vi "Test Component A Does Something.vi"(11 "Test Case In":refnum<class "Some Component A Test.lvclass">) -> (0 "error out":errorcluster, 3 "Test Case Out":refnum<class "Some Component A Test.lvclass">)   [LabVIEW 2020, in "Component A Test Suite.lvlib" / "Some Component A Test.lvclass"]
uses:
  Some Component A Test.lvclass
  Some Component A Test.lvclass/Some Component A Test.ctl
  b08caf3d-bad9-44fb-9ac4-9cc6f929a6d7.vi
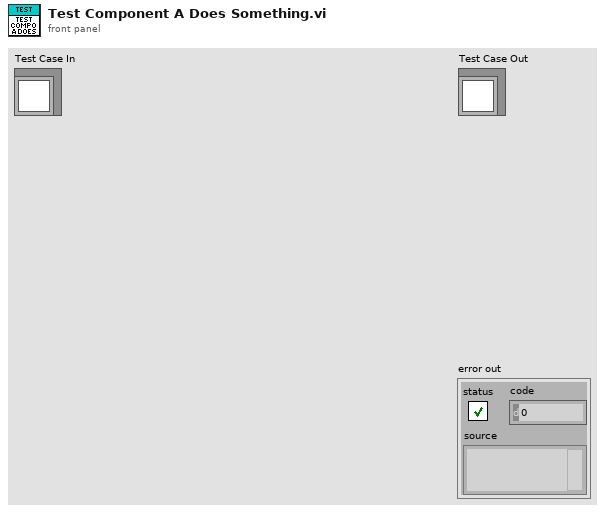
[diagram p1: front panel]
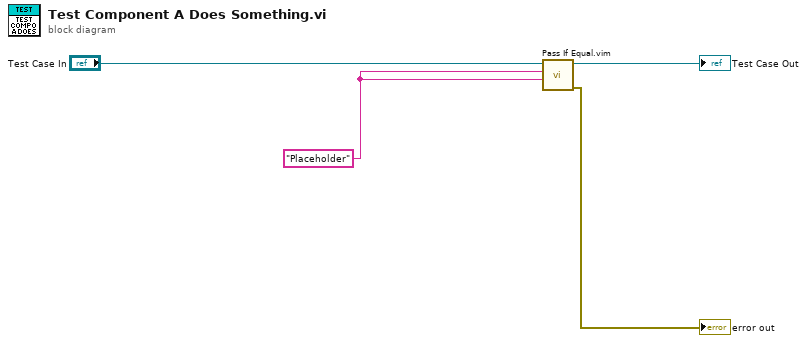
[diagram p0: block diagram]
diagram:
  w1 = "Placeholder"
  n1 = call "Pass If Equal.vim"("Actual"=w1, "Expected"=w1, "LUnit Test Case In"="Test Case In") -> ("error out"=→"error out":errorcluster, "LUnit Test Case Out"=→"Test Case Out":refnum<class "Some Component A Test.lvclass">)  [unwired: 7 in]
